vi "sortByChannelName.vi"(8 "error in (no error)":errorcluster, 10 "channelData in":T1(array[cluster]), 11 "ScriptEventList in":refnum<class "ScriptEventList.lvclass">) -> (0 "error out":errorcluster, 2 "channelData":T1(array[cluster]), 3 "ScriptEventList out":refnum<class "ScriptEventList.lvclass">)   [LabVIEW 2009, in "Tools.lvlib" / "Scripting.lvlib" / "ScriptEventList.lvclass"]
uses:
  ScriptEventList.lvclass
  DatabaseHelpers/Database Objects/Channel/Channel.lvclass
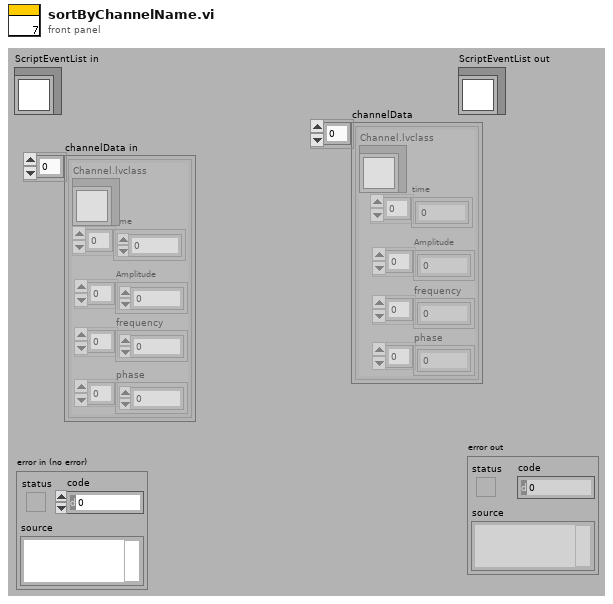
[diagram p1: front panel]
types:
  T1 = cluster{"Channel.lvclass":refnum<class "Channel.lvclass">, "time":dbl[], "Amplitude":dbl[], "frequency":dbl[], "phase":dbl[]}[]
  T2 = cluster{"Channel.lvclass":refnum<class "Channel.lvclass">, "time":dbl[], "Amplitude":dbl[], "frequency":dbl[], "phase":dbl[]}
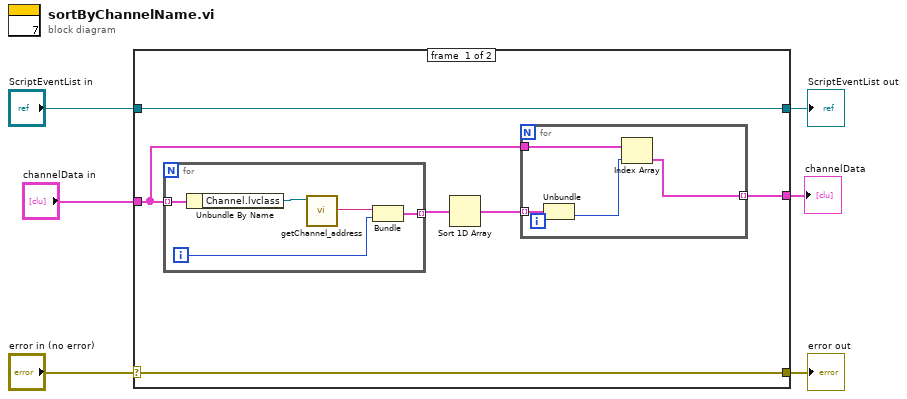
[diagram p0: block diagram]
diagram:
  n1 = case shown="No Error" "error in (no error)" {
    selector: "error in (no error)" -> [w11 w23]
    tunnel: [w11 w23] -> w5
    tunnel: [w12 w22] -> w3
    tunnel: "ScriptEventList in" -> [w12 w22]
    tunnel: "channelData in" -> [w8 _]
    tunnel: [w7 _] -> w1
    frame #0 {
      n2 = for {
        tunnel: w8 -> [w21] mode=indexing
        tunnel: [w17] -> w10 mode=indexing
        i -> [w18]
        n3 = Unbundle By Name(w21) -> ("Channel.lvclass"=w20:refnum<class "Channel.lvclass">)
        n4 = call "getChannel_address.vi"("Channel.lvclass in"=w20) -> ("channel_address"=w19:string)  [unwired: 8 in, 2 out]
        n5 = Bundle("channel_address"=w19, w18) -> (w17:cluster{"channel_address":string, i32})  [unwired: 1 in]
      }
      n6 = Sort 1D Array(array=w10) -> (sorted array=w9:cluster{"channel_address":string, i32}[])
      n7 = for {
        tunnel: w9 -> [w16] mode=indexing
        tunnel: w8 -> [w15]
        tunnel: [w13] -> w7 mode=indexing
        n8 = Unbundle(w16) -> (w14:i32)  [unwired: 1 out]
        n9 = Index Array(array=w15, index=w14) -> (element=w13:T2)
      }
    }
    frame #1 {
    }
  }
  "error out" <- w5
  "ScriptEventList out" <- w3
  "channelData" <- w1
